vi "Read DMA Number of Samples.vi"(8 "error in (no error)":errorcluster, 11 "Refs in":T1={"Data Type"=enum."Boolean", "DMA_SGL"=refnum, "DMA_U64"=refnum, "DMA_I64"=refnum, "DMA_FXP+/-32.8"=refnum, "DMA_FXP+/-64.32"=refnum, "DMA_U32"=refnum, "DMA_U16"=refnum, "DMA_U8"=refnum, "DMA_I32"=refnum, "DMA_I16"=refnum, "DMA_I8"=refnum, "DMA_FXP+/-32.16"=refnum} {"Data Type" format="%.0x"}) -> (0 "error out":errorcluster, 2 "Elements Remaining":u32, 3 "Refs out":T1={"Data Type"=enum."Boolean", "DMA_SGL"=refnum, "DMA_U64"=refnum, "DMA_I64"=refnum, "DMA_FXP+/-32.8"=refnum, "DMA_FXP+/-64.32"=refnum, "DMA_U32"=refnum, "DMA_U16"=refnum, "DMA_U8"=refnum, "DMA_I32"=refnum, "DMA_I16"=refnum, "DMA_I8"=refnum, "DMA_FXP+/-32.16"=refnum} {"Data Type" format="%.0x"})   [LabVIEW 2015, in "FPGA Addon Engine.lvlib"]
uses:
  FPGA Addon Engine.lvlib
  Types/DMA Input Refs.ctl
  Shared/Data Type.ctl
  <vilib>/rvi/errors/niLvFpgaAdjustHostInterfaceError.vi
  <vilib>/Utility/error.llb/Error Cluster From Error Code.vi
  <vilib>/rvi/interface/nirviMethod/nirviMethod.xnode
  <vilib>/FPGAPlugInAG/Dynamic/niLvFpga_ReadFifo_Dynamic.vi
  <vilib>/rvi/errors/niLvFpgaMergeErrorWithErrorCode.vi
  Shared/FPGA Addon Shared.lvlib
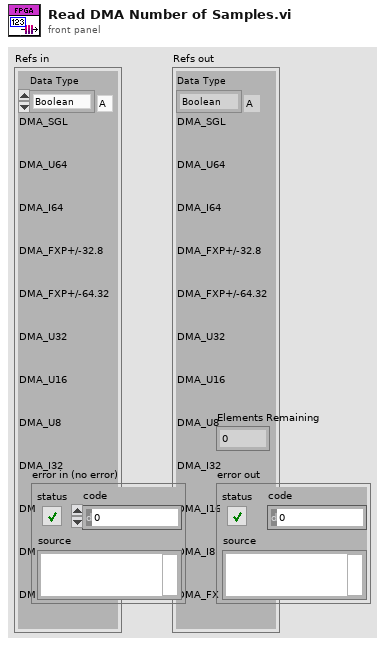
[diagram p1: front panel]
types:
  T1 = typedef "FPGA Addon Engine.lvlib/DMA Input Refs.ctl" = cluster{"Data Type":T2, "DMA_SGL":refnum<k20>, "DMA_U64":refnum<k20>, "DMA_I64":refnum<k20>, "DMA_FXP+/-32.8":refnum<k20>, "DMA_FXP+/-64.32":refnum<k20>, "DMA_U32":refnum<k20>, "DMA_U16":refnum<k20>, "DMA_U8":refnum<k20>, "DMA_I32":refnum<k20>, "DMA_I16":refnum<k20>, "DMA_I8":refnum<k20>, "DMA_FXP+/-32.16":refnum<k20>}
  T2 = typedef "FPGA Addon Shared.lvlib/Data Type.ctl" = enum8{"<Null>", "I8", "I16", "I32", "I64", "U8", "U16", "U32", "U64", "SGL", "Boolean", "Analog PWM In Settings", "Analog PWM In", "Digital PWM In Settings", "Digital PWM In", "Digital PWM Out", "Sine Out", "FXP+/-24.5", "FXP+/-16.5", "FXP+/-32.8", "FXP+/-64.32", "FXP+/-16.7", "FXP+/-20.5", "FXP+/-27.5", "FXP+/-32.16", "Digital Static In", "Digital Static Out", "Digital Static In Settings", "Digital WSS Out", "Quad Encoder Settings", "Quad Encoder In"}
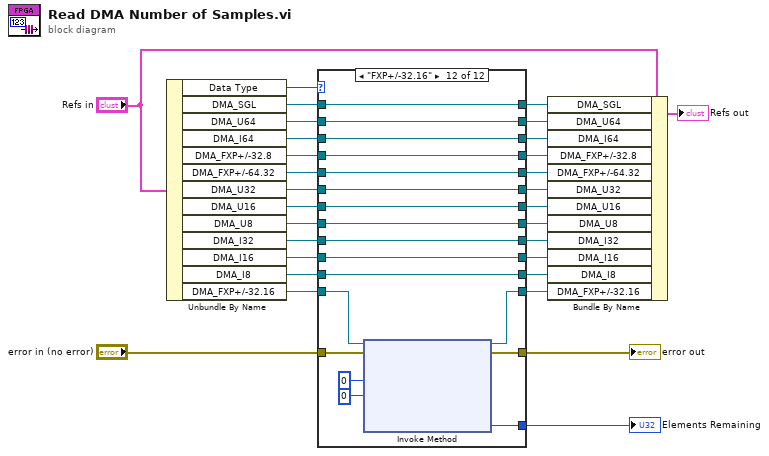
[diagram p0: block diagram]
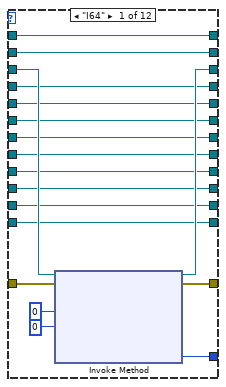
[diagram p2: hidden frame]
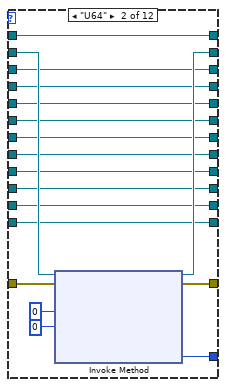
[diagram p3: hidden frame]
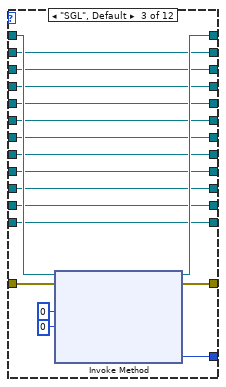
[diagram p4: hidden frame]
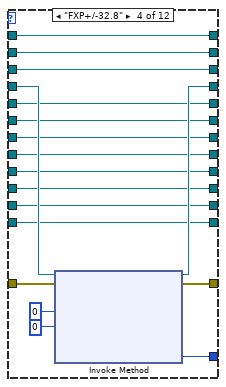
[diagram p5: hidden frame]
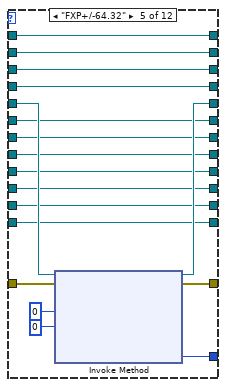
[diagram p6: hidden frame]
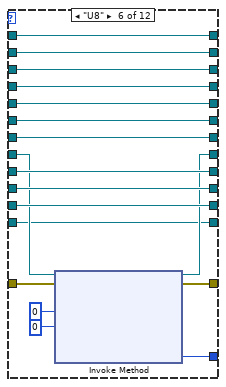
[diagram p7: hidden frame]
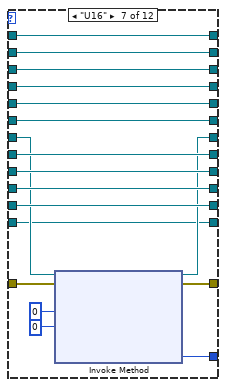
[diagram p8: hidden frame]
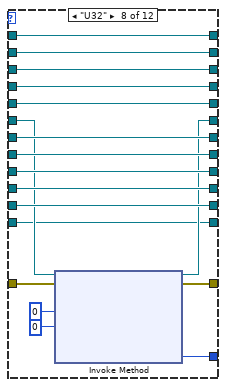
[diagram p9: hidden frame]
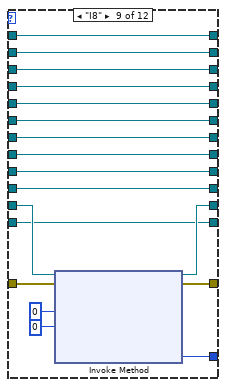
[diagram p10: hidden frame]
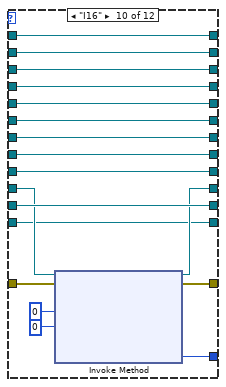
[diagram p11: hidden frame]
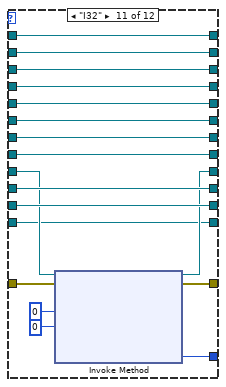
[diagram p12: hidden frame]
diagram:
  n1 = Unbundle By Name("Refs in") -> ("Data Type"=w24:T2, "DMA_SGL"=w25:refnum<k20>, "DMA_U64"=w26:refnum<k20>, "DMA_I64"=w20:refnum<k20>, "DMA_FXP+/-32.8"=w18:refnum<k20>, "DMA_FXP+/-64.32"=w16:refnum<k20>, "DMA_U32"=w3:refnum<k20>, "DMA_U16"=w5:refnum<k20>, "DMA_U8"=w7:refnum<k20>, "DMA_I32"=w9:refnum<k20>, "DMA_I16"=w11:refnum<k20>, "DMA_I8"=w13:refnum<k20>, "DMA_FXP+/-32.16"=w2:refnum<k20>)
  n2 = case shown="\"FXP+/-32.16\"" w24 {
    tunnel: "error in (no error)" -> [w48 w66 w84 w102 w120 w138 w156 w174 w192 w210 w228 w246]
    tunnel: [w43 w61 w83 w97 w115 w133 w151 w169 w187 w205 w223 w241] -> w29
    tunnel: [w47 w65 w82 w101 w119 w137 w155 w173 w191 w209 w227 w245] -> w22
    tunnel: [w46 w64 w81 w100 w118 w136 w154 w172 w190 w208 w226 w244] -> w23
    tunnel: w25 -> [w43 w61 w78 w97 w115 w133 w151 w169 w187 w205 w223 w241]
    tunnel: w26 -> [w41 w60 w77 w96 w110 w130 w148 w166 w184 w202 w220 w238]
    tunnel: [w41 w59 w77 w96 w110 w130 w148 w166 w184 w202 w220 w238] -> w30
    tunnel: w20 -> [w42 w58 w76 w94 w114 w132 w150 w168 w186 w204 w222 w240]
    tunnel: [w40 w58 w76 w94 w114 w132 w150 w168 w186 w204 w222 w240] -> w19
    tunnel: w18 -> [w39 w57 w75 w95 w113 w131 w149 w167 w185 w203 w221 w239]
    tunnel: [w39 w57 w75 w93 w113 w131 w149 w167 w185 w203 w221 w239] -> w17
    tunnel: w16 -> [w38 w56 w74 w92 w112 w124 w142 w160 w178 w196 w214 w232]
    tunnel: [w38 w56 w74 w92 w111 w124 w142 w160 w178 w196 w214 w232] -> w15
    tunnel: [w32 w50 w68 w86 w104 w125 w143 w161 w176 w197 w215 w233] -> w14
    tunnel: w13 -> [w32 w50 w68 w86 w104 w125 w143 w161 w177 w197 w215 w233]
    tunnel: [w33 w51 w69 w87 w105 w126 w144 w162 w179 w194 w216 w234] -> w12
    tunnel: w11 -> [w33 w51 w69 w87 w105 w126 w144 w162 w179 w195 w216 w234]
    tunnel: [w34 w52 w70 w88 w106 w127 w145 w163 w180 w198 w212 w230] -> w10
    tunnel: w9 -> [w34 w52 w70 w88 w106 w127 w145 w163 w180 w198 w213 w230]
    tunnel: [w35 w53 w71 w89 w107 w122 w146 w164 w181 w199 w217 w235] -> w8
    tunnel: w7 -> [w35 w53 w71 w89 w107 w123 w146 w164 w181 w199 w217 w235]
    tunnel: [w36 w54 w72 w90 w108 w128 w140 w165 w182 w200 w218 w236] -> w6
    tunnel: w5 -> [w36 w54 w72 w90 w108 w128 w141 w165 w182 w200 w218 w236]
    tunnel: [w37 w55 w73 w91 w109 w129 w147 w158 w183 w201 w219 w237] -> w4
    tunnel: w3 -> [w37 w55 w73 w91 w109 w129 w147 w159 w183 w201 w219 w237]
    tunnel: w2 -> [w31 w49 w67 w85 w103 w121 w139 w157 w175 w193 w211 w231]
    tunnel: [w31 w49 w67 w85 w103 w121 w139 w157 w175 w193 w211 w229] -> w1
    frame "I64" {
      n3 = xnode "Invoke Method"("FPGA VI Reference In"=w42, "error in"=w48, "Number of Elements"=u32 0, "Timeout (ms)"=0) -> ("FPGA VI Reference Out"=w40:refnum<k20>, "error out"=w47:errorcluster, "Elements Remaining"=w46:u32)  [unwired: 1 out]
    }
    frame "U64" {
      n4 = xnode "Invoke Method"("FPGA VI Reference In"=w60, "error in"=w66, "Number of Elements"=u32 0, "Timeout (ms)"=0) -> ("FPGA VI Reference Out"=w59:refnum<k20>, "error out"=w65:errorcluster, "Elements Remaining"=w64:u32)  [unwired: 1 out]
    }
    frame "SGL", Default {
      n5 = xnode "Invoke Method"("FPGA VI Reference In"=w78, "error in"=w84, "Number of Elements"=u32 0, "Timeout (ms)"=0) -> ("FPGA VI Reference Out"=w83:refnum<k20>, "error out"=w82:errorcluster, "Elements Remaining"=w81:u32)  [unwired: 1 out]
    }
    frame "FXP+/-32.8" {
      n6 = xnode "Invoke Method"("FPGA VI Reference In"=w95, "error in"=w102, "Number of Elements"=u32 0, "Timeout (ms)"=0) -> ("FPGA VI Reference Out"=w93:refnum<k20>, "error out"=w101:errorcluster, "Elements Remaining"=w100:u32)  [unwired: 1 out]
    }
    frame "FXP+/-64.32" {
      n7 = xnode "Invoke Method"("FPGA VI Reference In"=w112, "error in"=w120, "Number of Elements"=u32 0, "Timeout (ms)"=0) -> ("FPGA VI Reference Out"=w111:refnum<k20>, "error out"=w119:errorcluster, "Elements Remaining"=w118:u32)  [unwired: 1 out]
    }
    frame "U8" {
      n8 = xnode "Invoke Method"("FPGA VI Reference In"=w123, "error in"=w138, "Number of Elements"=u32 0, "Timeout (ms)"=0) -> ("FPGA VI Reference Out"=w122:refnum<k20>, "error out"=w137:errorcluster, "Elements Remaining"=w136:u32)  [unwired: 1 out]
    }
    frame "U16" {
      n9 = xnode "Invoke Method"("FPGA VI Reference In"=w141, "error in"=w156, "Number of Elements"=u32 0, "Timeout (ms)"=0) -> ("FPGA VI Reference Out"=w140:refnum<k20>, "error out"=w155:errorcluster, "Elements Remaining"=w154:u32)  [unwired: 1 out]
    }
    frame "U32" {
      n10 = xnode "Invoke Method"("FPGA VI Reference In"=w159, "error in"=w174, "Number of Elements"=u32 0, "Timeout (ms)"=0) -> ("FPGA VI Reference Out"=w158:refnum<k20>, "error out"=w173:errorcluster, "Elements Remaining"=w172:u32)  [unwired: 1 out]
    }
    frame "I8" {
      n11 = xnode "Invoke Method"("FPGA VI Reference In"=w177, "error in"=w192, "Number of Elements"=u32 0, "Timeout (ms)"=0) -> ("FPGA VI Reference Out"=w176:refnum<k20>, "error out"=w191:errorcluster, "Elements Remaining"=w190:u32)  [unwired: 1 out]
    }
    frame "I16" {
      n12 = xnode "Invoke Method"("FPGA VI Reference In"=w195, "error in"=w210, "Number of Elements"=u32 0, "Timeout (ms)"=0) -> ("FPGA VI Reference Out"=w194:refnum<k20>, "error out"=w209:errorcluster, "Elements Remaining"=w208:u32)  [unwired: 1 out]
    }
    frame "I32" {
      n13 = xnode "Invoke Method"("FPGA VI Reference In"=w213, "error in"=w228, "Number of Elements"=u32 0, "Timeout (ms)"=0) -> ("FPGA VI Reference Out"=w212:refnum<k20>, "error out"=w227:errorcluster, "Elements Remaining"=w226:u32)  [unwired: 1 out]
    }
    frame "FXP+/-32.16" {
      n14 = xnode "Invoke Method"("FPGA VI Reference In"=w231, "error in"=w246, "Number of Elements"=u32 0, "Timeout (ms)"=0) -> ("FPGA VI Reference Out"=w229:refnum<k20>, "error out"=w245:errorcluster, "Elements Remaining"=w244:u32)  [unwired: 1 out]
    }
  }
  "Elements Remaining" <- w23
  "error out" <- w22
  n15 = Bundle By Name(cluster="Refs in", "DMA_SGL"=w29, "DMA_U64"=w30, "DMA_I64"=w19, "DMA_FXP+/-32.8"=w17, "DMA_FXP+/-64.32"=w15, "DMA_U32"=w4, "DMA_U16"=w6, "DMA_U8"=w8, "DMA_I32"=w10, "DMA_I16"=w12, "DMA_I8"=w14, "DMA_FXP+/-32.16"=w1) -> (→"Refs out":T1)
